vi "Show Actors Core.vi"(8 "error in (no error)":errorcluster, 10 "Actor ID":string, 11 "Actor Monitor in":refnum<class "Actor Monitor.lvclass">) -> (0 "error out":errorcluster, 3 "Actor Monitor out":refnum<class "Actor Monitor.lvclass">)   [LabVIEW 2018, in "Monitored Actor.lvlib" / "Actor Monitor.lvclass"]
doc: "Opens a VI Server refence to the actor's core and opens it\n\nCopyright: MGI\nAuthored by: Derek Trepanier"
uses:
  Actor Monitor.lvclass
  UI Info.ctl
  Actor Monitor.lvclass/Actor Monitor.ctl
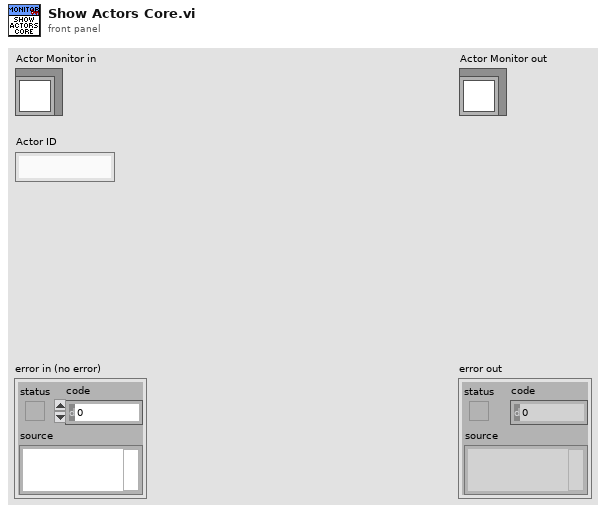
[diagram p1: front panel]
types:
  T1 = typedef "Monitored Actor.lvlib/Actor Monitor.lvclass/UI Info.ctl" = cluster{"Class Name":string, "Actor Core Name":string, "Ping Response Str":string}
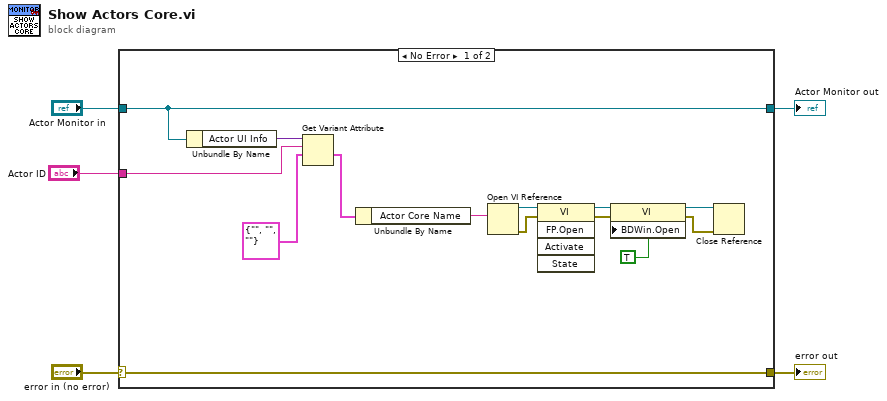
[diagram p0: block diagram]
diagram:
  n1 = case shown="No Error" "error in (no error)" {
    selector: "error in (no error)" -> [w19 w21]
    tunnel: [w19 w21] -> w4
    tunnel: [w18 w20] -> w2
    tunnel: "Actor Monitor in" -> [w18 w20]
    tunnel: "Actor ID" -> [w16 _]
    frame No Error {
      n2 = Unbundle By Name(w18) -> ("Actor UI Info"=w17:variant)
      n3 = Get Variant Attribute(Variant=w17, name=w16, default value (empty Variant)=T1 {"Class Name"="", "Actor Core Name"="", "Ping Response Str"=""} ("UI Info")) -> (value=w14:T1)  [unwired: 1 in, 3 out]
      n4 = Unbundle By Name(w14) -> ("Actor Core Name"=w6:string)
      n5 = Open VI Reference(vi path=w6) -> (vi reference=w13:refnum<vi>, error out=w9:errorcluster)  [unwired: 5 in]
      n6 = invoke class="VI" method="FP.Open"(reference=w13, error in=w9) -> (reference out=w12:refnum<vi>, error out=w8:errorcluster)  [unwired: 3 in, 3 out]
      n7 = property class="VI"(reference=w12, error in=w8, "BDWin.Open"=TRUE ("Block Diagram Window:Open")) -> (reference out=w10:refnum<vi>, error out=w7:errorcluster)
      n8 = Close Reference(reference=w10, error in (no error)=w7) -> ()  [unwired: 1 out]
    }
    frame Error {
    }
  }
  "error out" <- w4
  "Actor Monitor out" <- w2
